vi "AI Read Value.vi"(7 "ADC #":T1=-1, 8 "error in (no error)":errorcluster, 11 "VisaComms in":refnum<class "VisaComms.lvclass">) -> (0 "error out":errorcluster, 2 "Value":T2, 3 "VisaComms out":refnum<class "VisaComms.lvclass">)   [LabVIEW 2020, in "CTI.lvlib" / "VisaComms.lvclass"]
uses:
  VisaComms.lvclass
  Raw ADC.ctl
  ADC Number.ctl
  VisaComms.lvclass/VisaComms.ctl
  CTI.lvlib
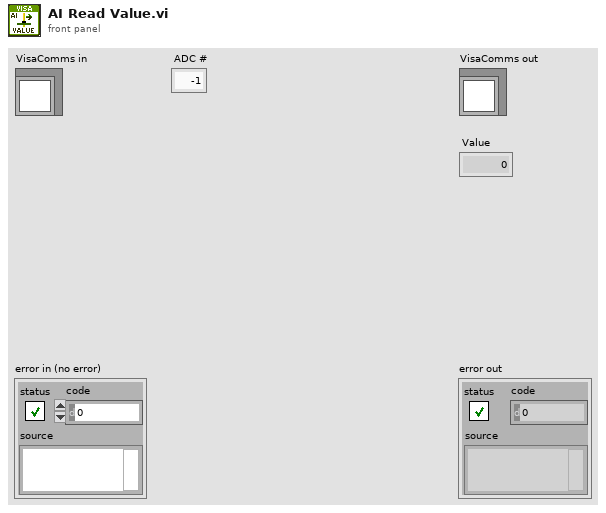
[diagram p1: front panel]
types:
  T1 = typedef "CTI.lvlib/ADC Number.ctl" = i8
  T2 = typedef "CTI.lvlib/Raw ADC.ctl" = u16
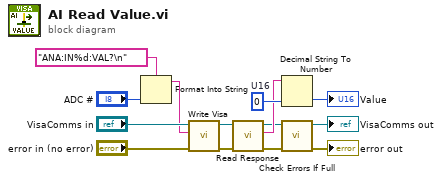
[diagram p0: block diagram]
diagram:
  w11 = u16 0  # U16
  n1 = Format Into String(format string="ANA:IN%d:VAL?\n", "ADC #") -> (resulting string=w3:string)  [unwired: 2 in, 1 out]
  n2 = call "Write Visa.vi"("error in (no error)"="error in (no error)", "write buffer"=w3, "VisaComms in"="VisaComms in") -> ("error out"=w1:errorcluster, "VisaComms out"=w2:refnum<class "VisaComms.lvclass">)  [unwired: 6 in, 1 out]
  n3 = call "Read Response.vi"("error in (no error)"=w1, "VisaComms in"=w2) -> ("error out"=w13:errorcluster, "Response"=w9:string, "VisaComms out"=w7:refnum<class "VisaComms.lvclass">)  [unwired: 7 in]
  n4 = Decimal String To Number(string=w9, default (0L)=w11) -> (number=→"Value":u16)  [unwired: 1 in, 1 out]
  n5 = call "Check Errors If Full.vi"("error in (no error)"=w13, "VisaComms in"=w7) -> ("error out"=→"error out":errorcluster, "VisaComms out"=→"VisaComms out":refnum<class "VisaComms.lvclass">)  [unwired: 8 in]
